vi "[GV]_PLATFORM Port NUM.vi"() -> ()   [LabVIEW 2016]
panel:
  in  "Platform port in":refnum<visa-resource-name>="COM6"
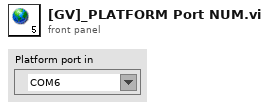
[diagram p1: front panel]
diagram:
